vi "Is CSM Module - ParseStateVI.vi"(8 "error in (no error)":errorcluster, 11 "Parse State VI Ref":refnum<vi>) -> (0 "error out":errorcluster, 2 "Is CSM Module?":bool, 3 "CSM Basic Refs":T1)   [LabVIEW 2017, in "CSM-Helper Utility.lvlib"]
doc: "#### Is CSM Module - ParseStateVI.vi\n\nDetermine if it is a CSM module through Parse State VI reference\n\n-- <b>Controls</b> --\n- <b>Parse State VI Ref</b>: Parse State VI reference\n\n-- <b>Indicators</b> --\n- <b>Is CSM Module?</b>: True If it is a CSM module\n- <b>CSM Basic Refs</b>: If This is a CSM module, It will return the basic references"
uses:
  CSM-Helper Utility.lvlib
  CSM Basic Refs.ctl
  CSM Module Type.ctl
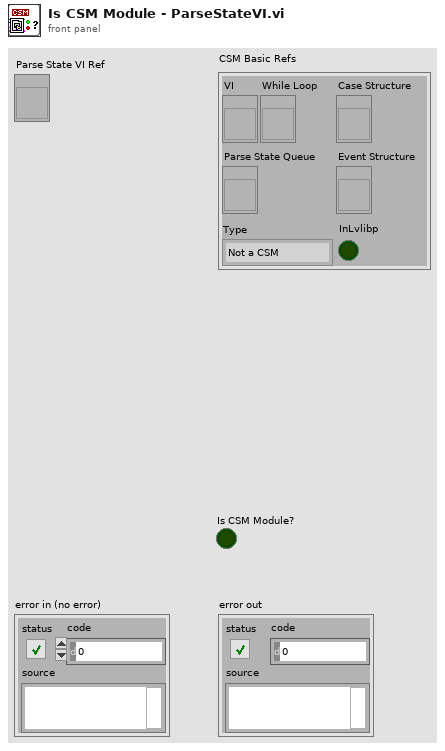
[diagram p1: front panel]
types:
  T1 = typedef "CSM-Helper Utility.lvlib/CSM Basic Refs.ctl" = cluster{"VI":refnum<vi>, "While Loop":refnum<vi>, "Case Structure":refnum<vi>, "Parse State Queue":refnum<vi>, "Event Structure":refnum<vi>, "Type":T2, "InLvlibp":bool}
  T2 = typedef "CSM-Helper Utility.lvlib/CSM Module Type.ctl" = enum16{"Not a CSM", "JKISM", "CSM"}
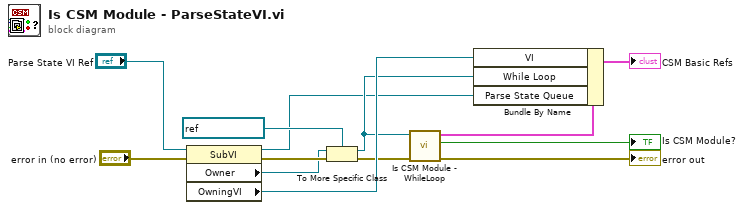
[diagram p0: block diagram]
diagram:
  n1 = property on="Property Node" class="SubVI"(reference="Parse State VI Ref", error in="error in (no error)") -> (reference out=w1:refnum<vi>, error out=w12:errorcluster, "Owner"=w8:refnum<vi>, "OwningVI"=w9:refnum<vi>)
  n2 = To More Specific Class(target class=refnum<vi> refnum ("WhileLoop"), reference=w8, error in=w12) -> (specific class reference=w5:refnum<vi>, error out=w6:errorcluster)
  n3 = call "Is CSM Module - WhileLoop.vi"("error in (no error)"=w6, "WhileLoop in"=w5) -> ("error out"=→"error out":errorcluster, "Is CSM Module?"=→"Is CSM Module?":bool, "CSM Basic Refs"=w2:T1)  [unwired: 6 in, 1 out]
  n4 = Bundle By Name(cluster=w2, "VI"=w9, "While Loop"=w5, "Parse State Queue"=w1) -> (→"CSM Basic Refs":T1)
